vi "Exit_prog.vi"(6 "EN/DIS":bool, 8 "error in (no error)":errorcluster, 9 "InputStr":string, 10 "Bytes to read":u32, 11 "USB Interface Name":refnum<visa-resource-name>="COM3") -> (1 "COMAND SET":bool, 2 "error out":errorcluster, 3 "RESET USB":bool)   [LabVIEW 2012]
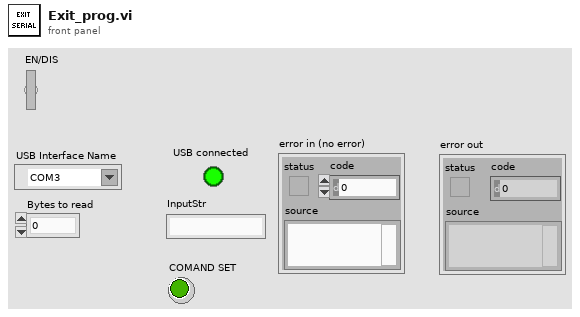
[diagram p1: front panel]
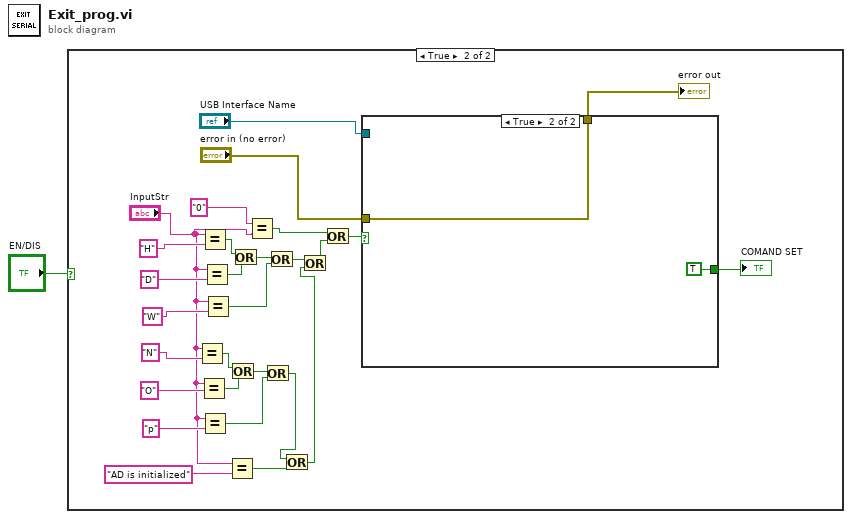
[diagram p0: block diagram]
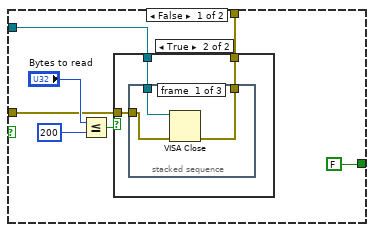
[diagram p3: hidden frame]
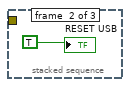
[diagram p5: hidden frame]
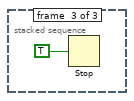
[diagram p6: hidden frame]
diagram:
  n1 = case shown="True" "EN/DIS" {
    frame False {
    }
    frame True {
      n2 = Equal?(x="InputStr", y="N") -> (x = y?=w17:bool)
      n3 = Equal?(x="InputStr", y="O") -> (x = y?=w18:bool)
      n4 = Equal?(x="InputStr", y="H") -> (x = y?=w23:bool)
      n5 = Equal?(x="InputStr", y="p") -> (x = y?=w11:bool)
      n6 = Equal?(x="InputStr", y="D") -> (x = y?=w24:bool)
      n7 = Equal?(x="InputStr", y="W") -> (x = y?=w21:bool)
      n8 = Equal?(x="InputStr", y="AD is initialized") -> (x = y?=w9:bool)
      n9 = Or(x=w17, y=w18) -> (x .or. y?=w12:bool)
      n10 = Or(x=w23, y=w24) -> (x .or. y?=w22:bool)
      n11 = Equal?(x="0", y="InputStr") -> (x = y?=w4:bool)
      n12 = Or(x=w12, y=w11) -> (x .or. y?=w8:bool)
      n13 = Or(x=w22, y=w21) -> (x .or. y?=w14:bool)
      n14 = Or(x=w8, y=w9) -> (x .or. y?=w7:bool)
      n15 = Or(x=w14, y=w7) -> (x .or. y?=w5:bool)
      n16 = Or(x=w4, y=w5) -> (x .or. y?=w6:bool)
      n17 = case shown="True" w6 {
        tunnel: "USB Interface Name" -> [w33 _]
        tunnel: "error in (no error)" -> [w32 w47]
        tunnel: [w31 w47] -> w26
        tunnel: [FALSE TRUE] -> w19
        frame False {
          n18 = Less Or Equal?(x="Bytes to read", y=200) -> (x <= y?=w36:bool)
          n19 = case shown="True" w36 {
            tunnel: [w37 w40] -> w31
            tunnel: w33 -> [_ w39]
            tunnel: w32 -> [w37 w38]
            frame False {
            }
            frame True {
              n20 = stacked-sequence {
                tunnel: [w43 _ _] -> w40
                tunnel: w39 -> [w42 _ _]
                tunnel: w38 -> [w41 _ _]
                frame #0 {
                  n21 = VISA Close(VISA resource name=w42, error in (no error)=w41) -> (error out=w43:errorcluster)
                }
                frame #1 {
                  "RESET USB" <- TRUE
                }
                frame #2 {
                  n22 = Stop(stop? (T)=TRUE ("Stop? (T)")) -> ()
                }
              }
            }
          }
        }
        frame True {
        }
      }
      "error out" <- w26
      "COMAND SET" <- w19
    }
  }
